vi "changeLaserFW.vi"(1 "FW pos":u8, 2 "inputFW":cluster{"FW Handle":u32, "init?":i16}, 3 "inputLaser":T1) -> (0 "changePos?":i16)   [LabVIEW 2015]
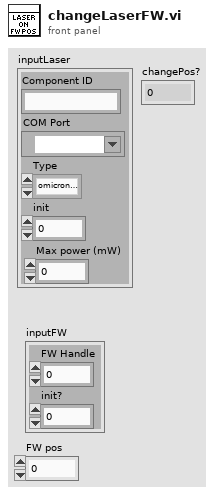
[diagram p1: front panel]
types:
  T1 = cluster{"Component ID":string, "COM Port":refnum<visa-resource-name>, "Type ":enum16{"omicronLuxX", "coherentObis"}, "init":i16, "Max power (mW)":dbl}
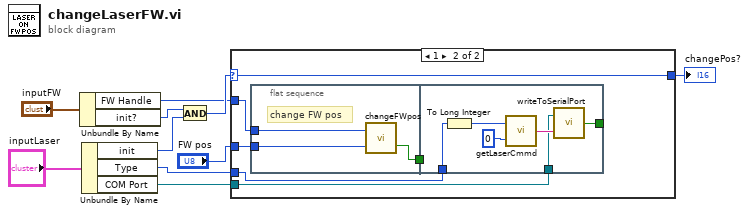
[diagram p0: block diagram]
diagram:
  n1 = Unbundle By Name("inputFW") -> ("FW Handle"=w4:u32, "init?"=w5:i16)
  n2 = Unbundle By Name("inputLaser") -> ("init"=w6:i16, "Type"=w3:enum16{"omicronLuxX", "coherentObis"}, "COM Port"=w2:refnum<visa-resource-name>)
  n3 = And(x=w5, y=w6) -> (x .and. y?=w8:i16)
  n4 = case shown="1" w8 {
    selector: w8 -> [w11 w12]
    tunnel: w4 -> [_ w17]
    tunnel: "FW pos" -> [_ w16]
    tunnel: w3 -> [_ w14]
    tunnel: w2 -> [_ w13]
    tunnel: [w11 w12] -> w1
    frame 0, Default {
    }
    frame 1 {
      n5 = flat-sequence {
        tunnel: w17 -> [w20]
        tunnel: w16 -> [w19]
        tunnel: [w18] -> w15
        tunnel: w15 -> [_]
        tunnel: w14 -> [w22]
        tunnel: w13 -> [w23]
        tunnel: [w21] -> _
        frame #0 {
          # "change FW pos"
          n6 = call "changeFWpos.vi"("FW pos"=w19, "FWhandle"=w20) -> ("fwPosChanged"=w18:bool)
        }
        frame #1 {
          n7 = To Long Integer(number=w22) -> (32bit integer=w24:i32)
          n8 = call "getLaserCmmd.vi"("Cmmd index"=0, "Laser type"=w24) -> ("Laser command"=w25:string)
          n9 = call "writeToSerialPort.vi"("Cmmd"=w25, "input COM Port"=w23) -> ("data written to port?"=w21:bool)
        }
      }
    }
  }
  "changePos?" <- w1
